vi "Pos2Dat.vi"(1 "Draw Area Size":T2, 2 "BCurvePosInPic":cluster{i16, i16}[](array[cluster]), 3 "GCurvePosInPic":cluster{i16, i16}[](array[cluster]), 4 "RCurvePosInPic":cluster{i16, i16}[](array[cluster])) -> (0 "FalseColorRatioData":T1)   [LabVIEW 2016]
uses:
  <vilib>/Utility/miscctls.llb/LVBoundsTypeDef.ctl
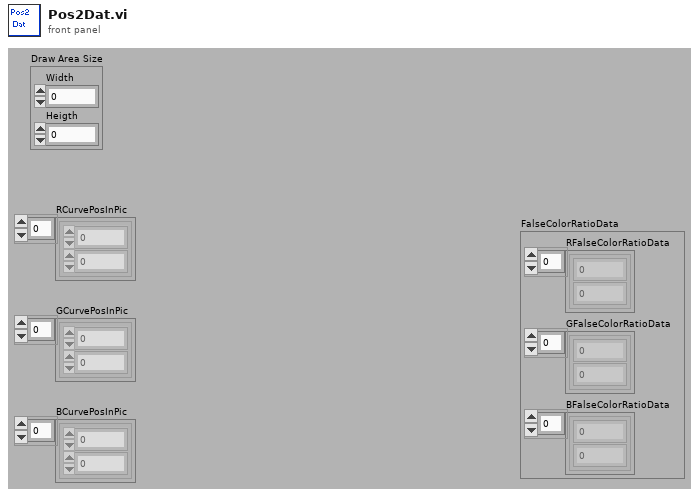
[diagram p1: front panel]
types:
  T1 = cluster{"RFalseColorRatioData":cluster{dbl, dbl}[], "GFalseColorRatioData":cluster{dbl, dbl}[], "BFalseColorRatioData":cluster{dbl, dbl}[]}
  T2 = typedef "LVBoundsTypeDef.ctl" = cluster{"Width":u32, "Height":u32}
  T3 = cluster{"FalseColorRatioData":cluster{dbl, dbl}[], "FalseColorRatioData":cluster{dbl, dbl}[], "FalseColorRatioData":cluster{dbl, dbl}[]}
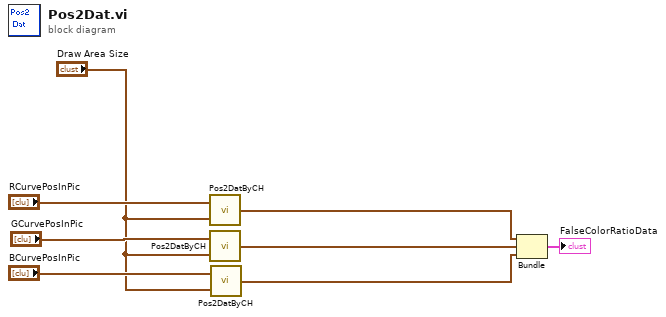
[diagram p0: block diagram]
diagram:
  n1 = call "Pos2DatByCH.vi"("Draw Area Size"="Draw Area Size", "PosInCurve"="RCurvePosInPic") -> ("FalseColorRatioData"=w4:cluster{dbl, dbl}[])
  n2 = call "Pos2DatByCH.vi"("Draw Area Size"="Draw Area Size", "PosInCurve"="GCurvePosInPic") -> ("FalseColorRatioData"=w3:cluster{dbl, dbl}[])
  n3 = call "Pos2DatByCH.vi"("Draw Area Size"="Draw Area Size", "PosInCurve"="BCurvePosInPic") -> ("FalseColorRatioData"=w2:cluster{dbl, dbl}[])
  n4 = Bundle("FalseColorRatioData"=w4, "FalseColorRatioData"=w3, "FalseColorRatioData"=w2) -> (→"FalseColorRatioData":T3)  [unwired: 1 out]
